vi "K2602 UpdateScript.vi"(8 "Script":string, 11 "Settings":T1={"Channel"=enum."Channel A", "Vset"=-1.0, "NPLC"=1.0, "I compliance"=0.001, "Repeat time"=3, "Delay ms"=500.0, "4-wire"=FALSE}) -> (3 "Output":string)   [LabVIEW 2012]
uses:
  SMU Settings.ctl
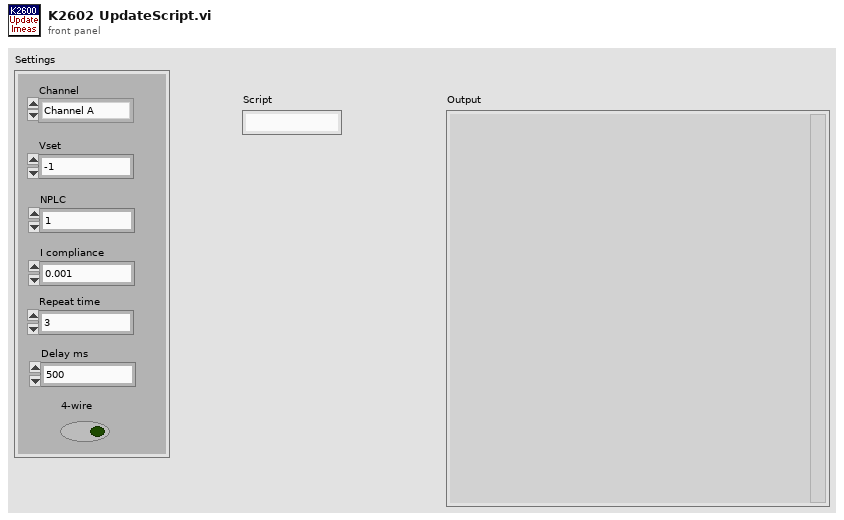
[diagram p1: front panel]
types:
  T1 = typedef "SMU Settings.ctl" = cluster{"Channel":enum32{"Channel A", "Channel B"}, "Vset":dbl, "NPLC":dbl, "I compliance":dbl, "Repeat time":u16, "Delay ms":dbl, "4-wire":bool}
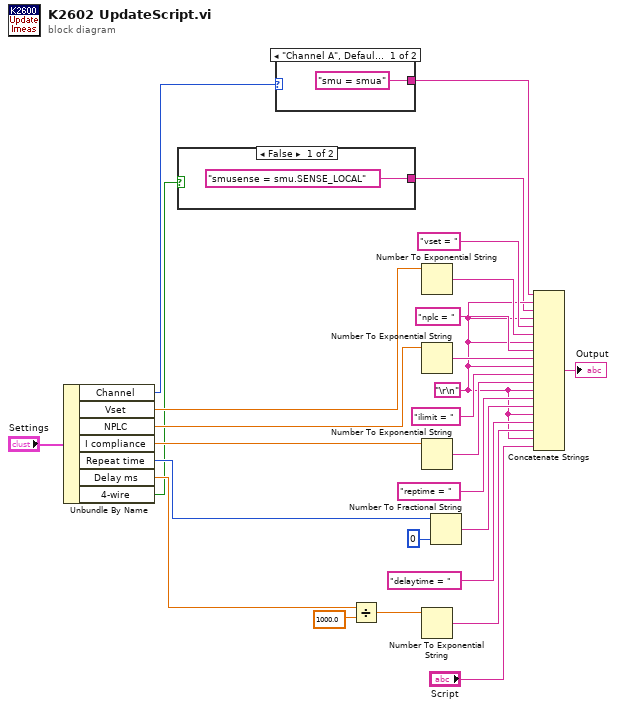
[diagram p0: block diagram]
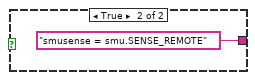
[diagram p2: hidden frame]
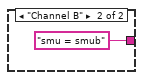
[diagram p3: hidden frame]
diagram:
  w2 = "\r\n"
  n1 = Unbundle By Name("Settings") -> ("Channel"=w25:enum32{"Channel A", "Channel B"}, "Vset"=w22:dbl, "NPLC"=w20:dbl, "I compliance"=w16:dbl, "Repeat time"=w9:u16, "Delay ms"=w6:dbl, "4-wire"=w3:bool)
  n2 = case shown="False" w3 {
    tunnel: ["smusense = smu.SENSE_LOCAL" "smusense = smu.SENSE_REMOTE"] -> w1
    frame False {
    }
    frame True {
    }
  }
  n3 = case shown="\"Channel A\", Default" w25 {
    tunnel: ["smu = smua" "smu = smub"] -> w24
    frame "Channel A", Default {
    }
    frame "Channel B" {
    }
  }
  n4 = Divide(x=w6, y=1000.0) -> (x/y=w4:dbl)
  n5 = Number To Exponential String(number=w22) -> (E-format string=w21:string)  [unwired: 3 in]
  n6 = Number To Exponential String(number=w20) -> (E-format string=w18:string)  [unwired: 3 in]
  n7 = Number To Exponential String(number=w16) -> (E-format string=w15:string)  [unwired: 3 in]
  n8 = Number To Exponential String(number=w4) -> (E-format string=w12:string)  [unwired: 3 in]
  n9 = Number To Fractional String(number=w9, precision (6)=i16 0) -> (F-format string=w8:string)  [unwired: 2 in]
  n10 = Concatenate Strings(w24, w2, w1, w2, "vset = ", w21, w2, "nplc = ", w18, w2, "ilimit = ", w15, w2, "reptime = ", w8, w2, "delaytime = ", w12, w2, "Script") -> (→"Output":string)
